vi "Partcalpm Control&FB.vi"(10 "Enum":T1(ring)) -> (2 "Part UnClamp Feedback":bool, 3 "Part Clamp Feedback":bool)   [LabVIEW 2015]
uses:
  Galobal variable_TI.vi
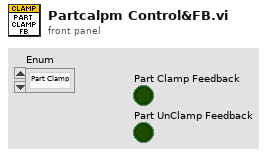
[diagram p1: front panel]
types:
  T1 = enum16{"Part Clamp", "Part Unclamp", "Part Clamp Input Check", "Part Unclamp Input Check"}
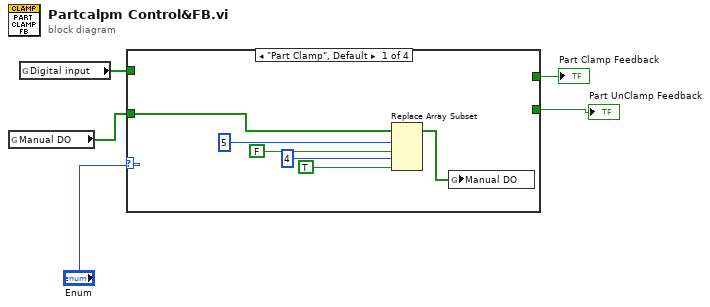
[diagram p0: block diagram]
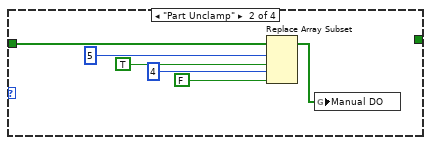
[diagram p2: hidden frame]
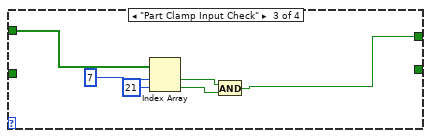
[diagram p3: hidden frame]
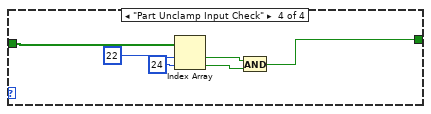
[diagram p4: hidden frame]
diagram:
  n1 = global read "Galobal variable_TI.vi" "Manual DO"() -> (w1:bool[])
  n2 = global read "Galobal variable_TI.vi" "Digital input"() -> (w4:bool[])
  n3 = case shown="\"Part Clamp\", Default" "Enum" {
    tunnel: w1 -> [w7 w13 _ w25]
    tunnel: w4 -> [_ _ w23 _]
    tunnel: [_ _ w18 _] -> w3
    tunnel: [_ _ _ w24] -> w2
    frame "Part Clamp", Default {
      n4 = Replace Array Subset(array=w7, new element #1=FALSE ("new element/subarray"), index #1=5 ("index"), new element #2=TRUE ("new element/subarray"), index #2=4 ("index")) -> (w6:bool[])
      n5 = global write "Galobal variable_TI.vi" "Manual DO"(w6) -> ()
    }
    frame "Part Unclamp" {
      n6 = Replace Array Subset(array=w13, new element #1=TRUE ("new element/subarray"), index #1=5 ("index"), new element #2=FALSE ("new element/subarray"), index #2=4 ("index")) -> (w12:bool[])
      n7 = global write "Galobal variable_TI.vi" "Manual DO"(w12) -> ()
    }
    frame "Part Clamp Input Check" {
      n8 = Index Array(array=w23, index #1=7 ("index"), index #2=21 ("index")) -> (element #1=w20:bool, element #2=w19:bool)
      n9 = And(x=w20, y=w19) -> (x .and. y?=w18:bool)
    }
    frame "Part Unclamp Input Check" {
      n10 = Index Array(array=w25, index #1=22 ("index"), index #2=24 ("index")) -> (element #1=w27:bool, element #2=w26:bool)
      n11 = And(x=w27, y=w26) -> (x .and. y?=w24:bool)
    }
  }
  "Part Clamp Feedback" <- w3
  "Part UnClamp Feedback" <- w2
